vi "uc480_SubVI_Example_Timing.vi"(0 ".NET (Reference)":refnum<k24>, 5 "Pixelclock":i32, 7 "Exposure time":dbl, 9 "Framerate":dbl, 11 "Error In":errorcluster) -> (6 "Pixelclock":i32, 8 "Exposure time":dbl, 10 "Framerate":dbl, 15 "Error Out":errorcluster)   [LabVIEW 2018]
uses:
  C:/Users/user/Desktop/Thorcam/uc480DotNet.dll
  uc480DotNet.dll
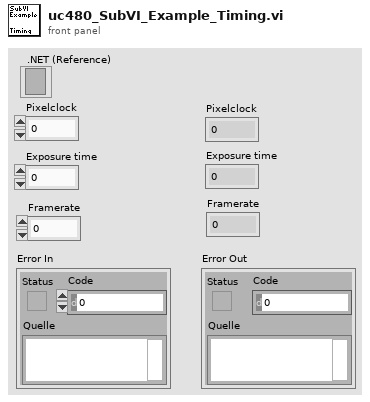
[diagram p1: front panel]
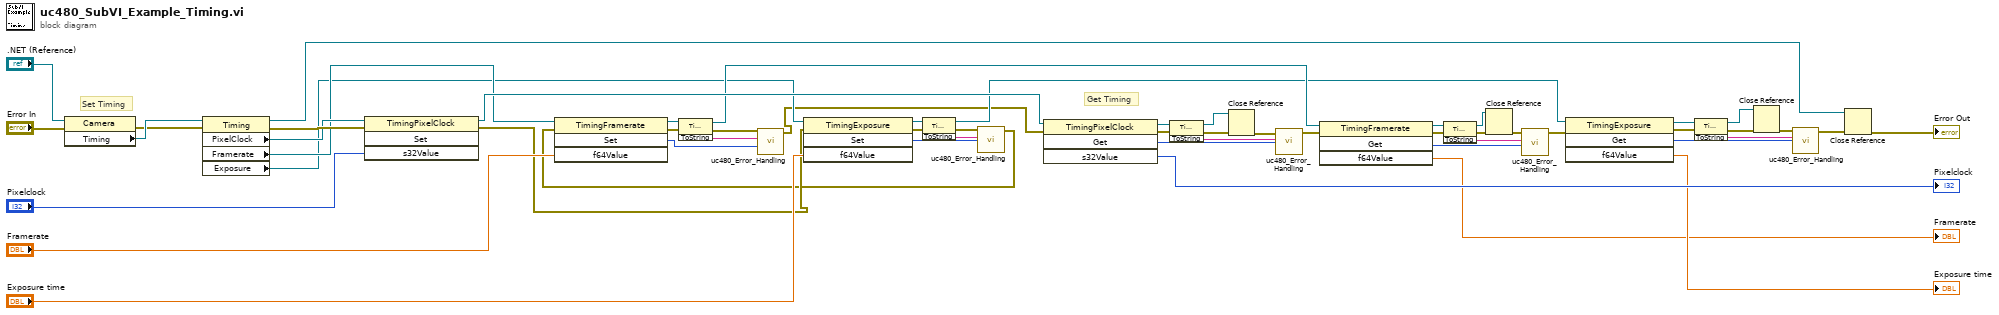
[diagram p0: block diagram]
diagram:
  # "Get Timing"
  # "Set Timing"
  n1 = property class="Camera"(reference=".NET (Reference)", error in="Error In") -> (error out=w1:errorcluster, "Timing"=w44:refnum<k24>)  [unwired: 1 out]
  n2 = property class="Timing"(reference=w44, error in=w1) -> (reference out=w11:refnum<k24>, error out=w16:errorcluster, "PixelClock"=w10:refnum<k24>, "Framerate"=w8:refnum<k24>, "Exposure"=w6:refnum<k24>)
  n3 = invoke class="TimingPixelClock" method="Set"(reference=w10, error in=w16, "s32Value"="Pixelclock") -> (reference out=w9:refnum<k24>, error out=w4:errorcluster)  [unwired: 1 in, 2 out]
  n4 = invoke class="TimingExposure" method="Set"(reference=w6, error in=w4, "f64Value"="Exposure time") -> (reference out=w47:refnum<k24>, error out=w48:errorcluster, "Set"=w49:i32)  [unwired: 1 in, 1 out]
  n5 = invoke class="TimingExposure" method="ToString"(reference=w47, error in=w48) -> (reference out=w5:refnum<k24>, error out=w14:errorcluster, "ToString"=w50:string)  [unwired: 1 in]
  n6 = call "uc480_Error_Handling.vi"("Error Code"=w49, "Error String"=w50, "Error In"=w14) -> ("Error Out"=w3:errorcluster)  [unwired: 8 in]
  n7 = invoke on="Methodenknoten" class="TimingFramerate" method="Set"(reference=w8, error in=w3, "f64Value"="Framerate") -> (reference out=w56:refnum<k24>, error out=w55:errorcluster, "Set"=w54:i32)  [unwired: 1 in, 1 out]
  n8 = invoke class="TimingFramerate" method="ToString"(reference=w56, error in=w55) -> (reference out=w7:refnum<k24>, error out=w15:errorcluster, "ToString"=w53:string)  [unwired: 1 in]
  n9 = call "uc480_Error_Handling.vi"("Error Code"=w54, "Error String"=w53, "Error In"=w15) -> ("Error Out"=w2:errorcluster)  [unwired: 8 in]
  n10 = invoke class="TimingPixelClock" method="Get"(reference=w9, error in=w2) -> (reference out=w41:refnum<k24>, error out=w40:errorcluster, "Get"=w38:i32, "s32Value"=→"Pixelclock":i32)  [unwired: 2 in]
  n11 = invoke class="TimingPixelClock" method="ToString"(reference=w41, error in=w40) -> (reference out=w17:refnum<k24>, error out=w19:errorcluster, "ToString"=w39:string)  [unwired: 1 in]
  n12 = Close Reference(reference=w17, error in (no error)=w19) -> (error out=w18:errorcluster)
  n13 = call "uc480_Error_Handling.vi"("Error Code"=w38, "Error String"=w39, "Error In"=w18) -> ("Error Out"=w29:errorcluster)  [unwired: 8 in]
  n14 = invoke class="TimingFramerate" method="Get"(reference=w7, error in=w29) -> (reference out=w37:refnum<k24>, error out=w36:errorcluster, "Get"=w34:i32, "f64Value"=→"Framerate":dbl)  [unwired: 2 in]
  n15 = invoke class="TimingFramerate" method="ToString"(reference=w37, error in=w36) -> (reference out=w20:refnum<k24>, error out=w22:errorcluster, "ToString"=w35:string)  [unwired: 1 in]
  n16 = Close Reference(reference=w20, error in (no error)=w22) -> (error out=w21:errorcluster)
  n17 = call "uc480_Error_Handling.vi"("Error Code"=w34, "Error String"=w35, "Error In"=w21) -> ("Error Out"=w28:errorcluster)  [unwired: 8 in]
  n18 = invoke class="TimingExposure" method="Get"(reference=w5, error in=w28) -> (reference out=w33:refnum<k24>, error out=w32:errorcluster, "Get"=w30:i32, "f64Value"=→"Exposure time":dbl)  [unwired: 2 in]
  n19 = invoke class="TimingExposure" method="ToString"(reference=w33, error in=w32) -> (reference out=w25:refnum<k24>, error out=w24:errorcluster, "ToString"=w31:string)  [unwired: 1 in]
  n20 = Close Reference(reference=w25, error in (no error)=w24) -> (error out=w23:errorcluster)
  n21 = call "uc480_Error_Handling.vi"("Error Code"=w30, "Error String"=w31, "Error In"=w23) -> ("Error Out"=w13:errorcluster)  [unwired: 8 in]
  n22 = Close Reference(reference=w11, error in (no error)=w13) -> (error out=→"Error Out":errorcluster)
